vi "ErrorPostRun.vi"(8 "error in (no error)":errorcluster) -> (0 "error out":errorcluster)   [LabVIEW 2017, in "ErrorMonitor.lvlib"]
doc: "This VI releases the Error Module queue."
uses:
  ErrorMonitor.lvlib
  Queue/TypeDefs/queueFGVState.ctl
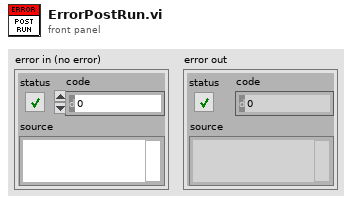
[diagram p1: front panel]
types:
  T1 = typedef "ErrorMonitor.lvlib/queueFGVState.ctl" = enum16{"set", "get"}
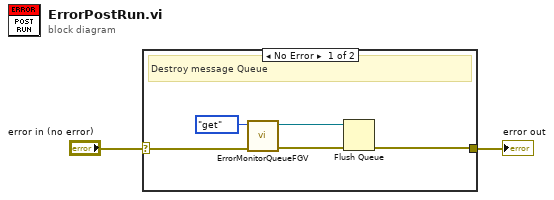
[diagram p0: block diagram]
diagram:
  n1 = case shown="No Error" "error in (no error)" {
    selector: "error in (no error)" -> [w7 w8]
    tunnel: [w3 w8] -> w1
    frame No Error {
      # "Destroy message Queue"
      n2 = call "ErrorMonitorQueueFGV.vi"("error in (no error)"=w7, 11:queueFGVState."get") -> ("error out"=w5:errorcluster, "queue out"=w4:refnum<queue>)  [unwired: 8 in]
      n3 = Flush Queue(queue=w4, error in (no error)=w5) -> (error out=w3:errorcluster)  [unwired: 2 out]
    }
    frame Error {
    }
  }
  "error out" <- w1
